vi "绘制选中框.vi"(8 "error in (no error)":errorcluster caption="错误输入（无错误）", 11 "程序 输入":refnum<class "程序.lvclass">) -> (0 "error out":errorcluster caption="错误输出", 3 "程序 输出":refnum<class "程序.lvclass">)   [LabVIEW 2018, in "程序.lvclass"]
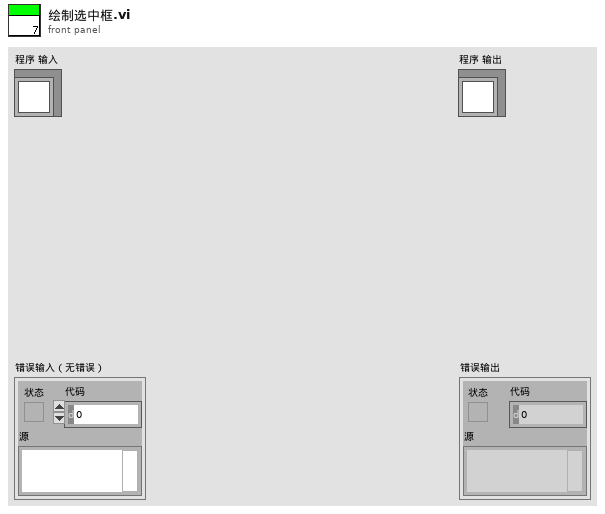
[diagram p1: front panel]
types:
  T1 = cluster{"Width":i16, "Style":enum32{"Solid", "Dash", "Dot", "DashDot", "DashDotDot"}}
  T2 = typedef "LVBoundsTypeDef.ctl" = cluster{"Width":u32, "Height":u32}
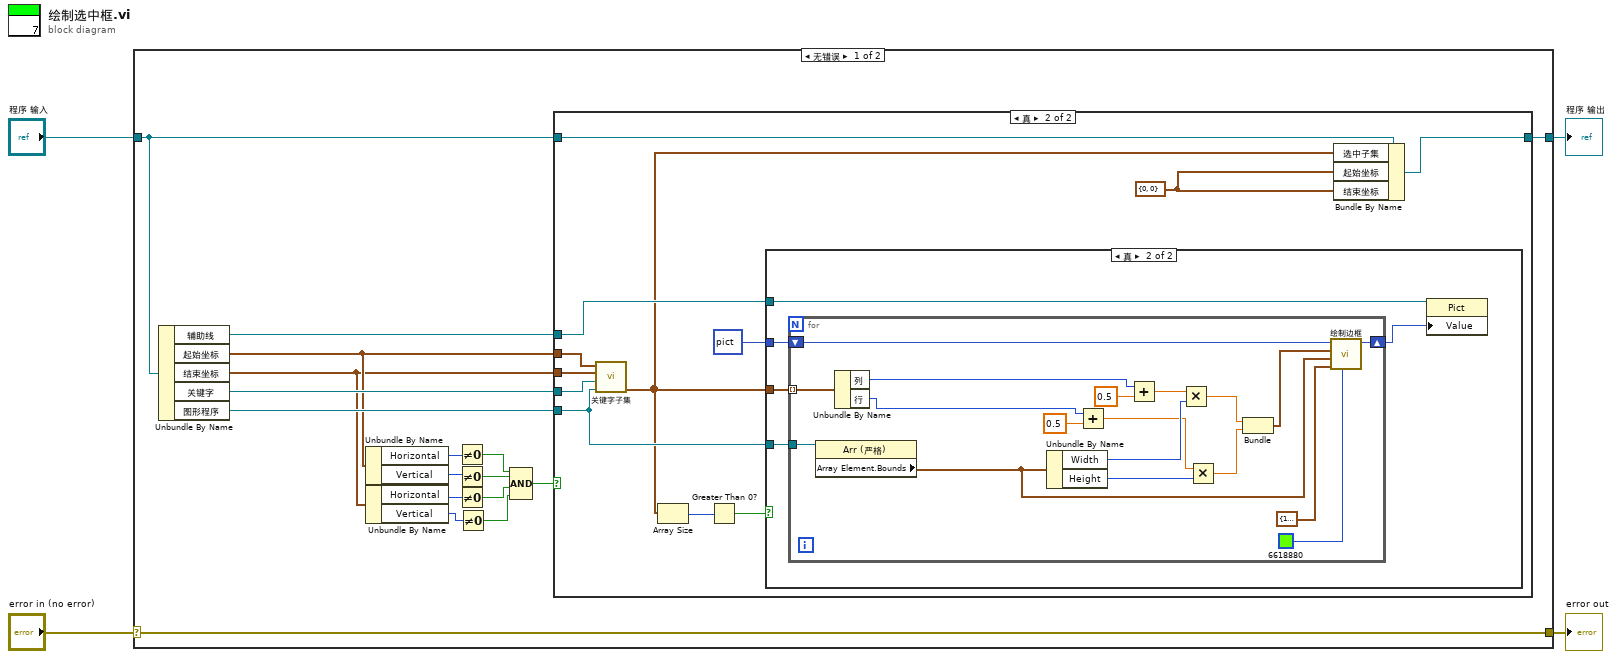
[diagram p0: block diagram]
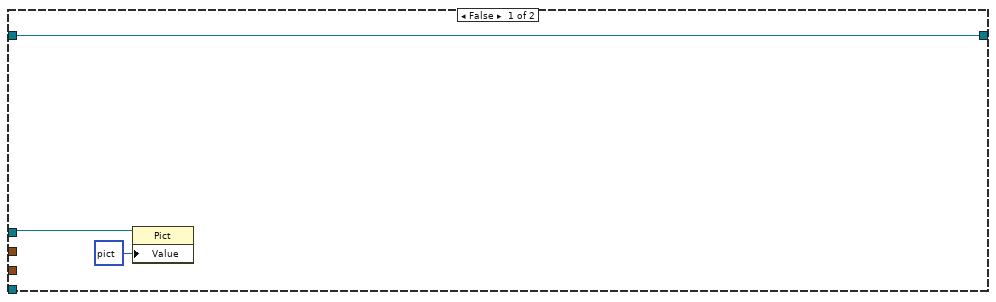
[diagram p2: hidden frame]
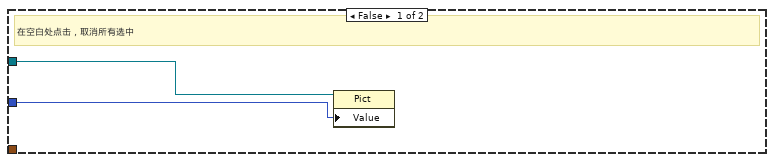
[diagram p3: hidden frame]
diagram:
  n1 = case shown="无错误" "error in (no error)" {
    selector: "error in (no error)" -> [w21 w63]
    tunnel: [w21 w63] -> w3
    tunnel: [w14 w62] -> w1
    tunnel: "程序 输入" -> [w15 w62]
    frame No Error {
      n2 = Unbundle By Name(w15) -> ("辅助线"=w20:refnum<vi>, "起始坐标"=w17:cluster{"Horizontal":i32, "Vertical":i32}, "结束坐标"=w16:cluster{"Horizontal":i32, "Vertical":i32}, "关键字"=w19:refnum<vi>, "图形程序"=w18:refnum<vi>)
      n3 = Unbundle By Name(w17) -> ("Horizontal"=w13:i32, "Vertical"=w12:i32)
      n4 = Unbundle By Name(w16) -> ("Horizontal"=w11:i32, "Vertical"=w10:i32)
      n5 = Not Equal To 0?(x=w13) -> (x != 0?=w9:bool)
      n6 = Not Equal To 0?(x=w12) -> (x != 0?=w8:bool)
      n7 = Not Equal To 0?(x=w11) -> (x != 0?=w7:bool)
      n8 = Not Equal To 0?(x=w10) -> (x != 0?=w6:bool)
      n9 = Compound Arithmetic op=AND ("复合运算")(w9, w8, w7, w6) -> (w5:bool)
      n10 = case shown="真" w5 {
        tunnel: w20 -> [w23 w33]
        tunnel: w17 -> [_ w32]
        tunnel: w16 -> [_ w31]
        tunnel: w19 -> [_ w30]
        tunnel: w18 -> [_ w29]
        tunnel: w15 -> [w24 w27]
        tunnel: [w24 w26] -> w14
        frame False {
          n11 = property class="Pict"(reference=w23, "Value"=picture data[5B] ("值")) -> ()  [unwired: 1 in, 2 out]
        }
        frame True {
          w28 = cluster{"Horizontal":i32, "Vertical":i32} {"Horizontal"=0, "Vertical"=0} ("起始坐标")
          n12 = call "关键字子集.vi"("图形程序"=w29, "关键字"=w30, "结束坐标"=w31, "起始坐标"=w32) -> ("选中子集"=w25:cluster{"行":i32, "列":i32}[])  [unwired: 7 in]
          n13 = Array Size(array=w25) -> (size(s)=w34:i32)
          n14 = Greater Than 0?(x=w34) -> (x > 0?=w35:bool)
          n15 = case shown="真" w35 {
            tunnel: w25 -> [_ w43]
            tunnel: w29 -> [_ w42]
            tunnel: w33 -> [w38 w40]
            tunnel: picture data[5B] ("new picture") -> [w37 w41]
            frame False {
              # "在空白处点击，取消所有选中"
              n16 = property class="Pict"(reference=w38, "Value"=w37) -> ()  [unwired: 1 in, 2 out]
            }
            frame True {
              n17 = for {
                shift-right: [w46] -> w39
                shift-left: w41 -> [w47]
                tunnel: w43 -> [w49] mode=indexing
                tunnel: w42 -> [w48]
                n18 = property class="Arr (严格)"(reference=w48) -> ("Array Element.Bounds"=w44:T2)  [unwired: 1 in, 2 out]
                n19 = Unbundle By Name(w49) -> ("列"=w51:i32, "行"=w50:i32)
                n20 = Unbundle By Name(w44) -> ("Width"=w60:u32, "Height"=w61:u32)
                n21 = Add(x=w50, y=0.5) -> (x+y=w56:dbl)
                n22 = Add(x=w51, y=0.5) -> (x+y=w59:dbl)
                n23 = Multiply(x=w59, y=w60) -> (x*y=w55:dbl)
                n24 = Multiply(x=w56, y=w61) -> (x*y=w54:dbl)
                n25 = Bundle(w55, w54) -> (w45:cluster{dbl, dbl})  [unwired: 1 in]
                n26 = call "绘制边框.vi"("颜色"=u32 6618880, "画笔"=T1 {"Width"=1, "Style"=enum."Dot"}, "大小"=w44, "中心"=w45, "picture"=w47) -> ("new picture"=w46:picture)  [unwired: 6 in]
              }
              n27 = property class="Pict"(reference=w40, "Value"=w39) -> ()  [unwired: 1 in, 2 out]
            }
          }
          n28 = Bundle By Name(cluster=w27, "选中子集"=w25, "起始坐标"=w28, "结束坐标"=w28) -> (w26:refnum<class "程序.lvclass">)
        }
      }
    }
    frame Error {
    }
  }
  "error out" <- w3
  "程序 输出" <- w1
